vi "Model Initial Values - Add Models RTM Dependency.vi"(8 "error in (no error)":errorcluster, 9 "Menu hierarchy in":string[](array[string]), 11 "Node Ptr":u64 format="%.0x") -> (0 "error out":errorcluster, 1 "Menu hierarchy out":string[](array[string]), 3 "Action":T1)   [LabVIEW 2011, in "Model Initial Values Custom Device.lvlib"]
uses:
  Model Initial Values Custom Device.lvlib
  <vilib>/NI Veristand/Custom Device API/Custom Device RTM Dependency.ctl
  Model Initial Values - Global.vi
  <vilib>/NI Veristand/Custom Device API/Get Item Property (Dependent Node Pointer).vi
  <vilib>/NI Veristand/Custom Device API/Custom Device API.lvlib
  <vilib>/NI Veristand/Custom Device Tools/Custom Device Utility Library/Custom Device Utility Library.lvlib
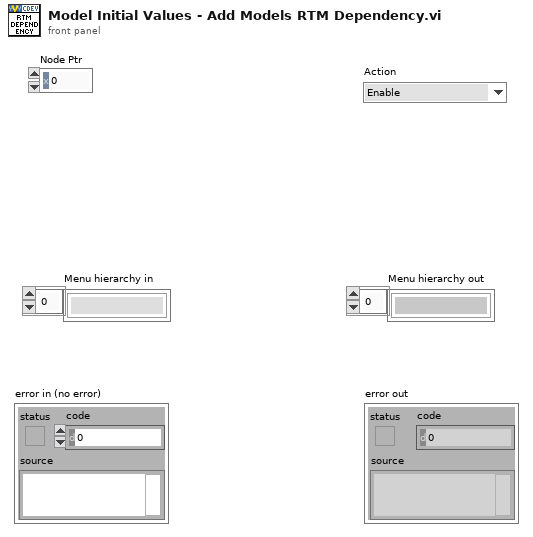
[diagram p1: front panel]
types:
  T1 = typedef "Custom Device API.lvlib/Custom Device RTM Dependency.ctl" = enum16{"Enable", "Disable", "Hide"}
  T2 = typedef "Custom Device API.lvlib/Custom Device Item Ref.ctl" = u64
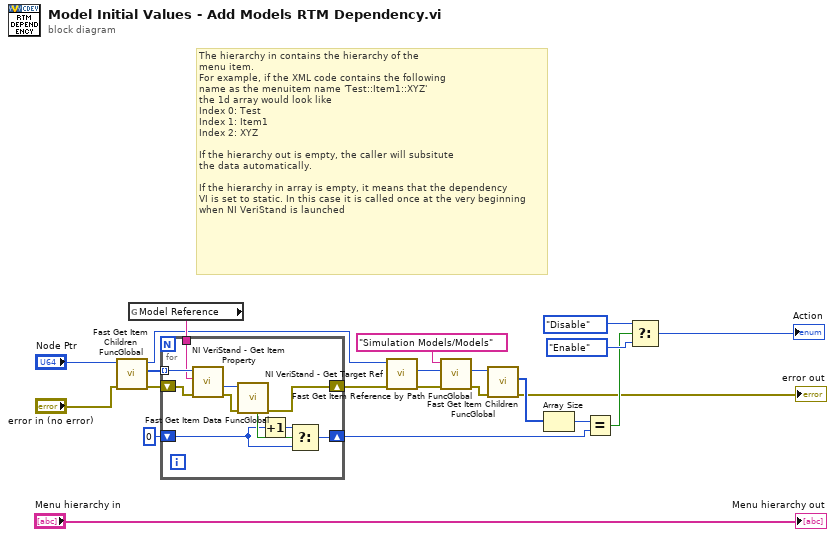
[diagram p0: block diagram]
diagram:
  # "The hierarchy in contains the hierarchy of the\nmenu item.\nFor example, if the XML code contains the following\nname as the menuitem name 'Test::Item1::XYZ'\nthe 1d array would look like\nIndex 0: Test\nIndex 1: Item1\nIndex 2: XYZ\n\nIf the hierarchy out is empty, the caller will subsitute\nthe data automatically.\n\nIf the hierarchy in array is empty, it means that the dependency\nVI is set to static. In this case it is called once at the very beginning\nwhen NI VeriStand is launched"
  n1 = call "Fast Get Item Children FuncGlobal.vi"("error in (no error)"="error in (no error)", "Item Ref in"="Node Ptr") -> ("error out"=w15:errorcluster, "Child Refs"=w16:T2[], "Item Ref out"=w8:T2)  [unwired: 6 in, 1 out]
  n2 = global read "Model Initial Values - Global.vi" "Model Reference"() -> (w14:string)
  n3 = for {
    tunnel: w16 -> [w31] mode=indexing
    shift-right: [w23] -> w9
    shift-left: w15 -> [w29]
    tunnel: w14 -> [w28]
    shift-right: [w25] -> w3
    shift-left: 0 -> [w24]
    n4 = call-poly <vilib>:"NI VeriStand - Get Item Property.vi"("error in (no error)"=w29, "Property Name"=w28, "Item Ref in"=w31) -> ("error out"=w30:errorcluster, "Dependent Node Ref"=w32:T2)  [unwired: 5 in, 2 out]
    n5 = call "Fast Get Item Data FuncGlobal.vi"("error in (no error)"=w30, "Item Ref in"=w32) -> ("error out"=w23:errorcluster, "Found"=w26:bool)  [unwired: 6 in, 2 out]
    n6 = Increment(x=w24) -> (x+1=w27:i32)
    n7 = Select(t=w27, s=w26, f=w24) -> (s? t:f=w25:i32)
  }
  n8 = call <vilib>:"NI VeriStand - Get Target Ref.vi"("error in"=w9, "Item Ref in"=w8) -> ("error out"=w10:errorcluster, "Target Ref"=w12:T2)  [unwired: 6 in, 2 out]
  n9 = call "Fast Get Item Reference by Path FuncGlobal.vi"("error in (no error)"=w10, "Root Ref"=w12, "Item Path in"="Simulation Models/Models" ("Relative Item Path")) -> ("error out"=w6:errorcluster, "Item Ref"=w7:T2)  [unwired: 5 in, 2 out]
  n10 = call "Fast Get Item Children FuncGlobal.vi"("error in (no error)"=w6, "Item Ref in"=w7) -> ("error out"=→"error out":errorcluster, "Child Refs"=w5:T2[])  [unwired: 6 in, 2 out]
  n11 = Array Size(array=w5) -> (size(s)=w4:i32)
  n12 = Equal?(x=w4, y=w3) -> (x = y?=w2:bool)
  n13 = Select(t=Custom_Device_RTM_Dependency."Disable" ("Action"), s=w2, f=Custom_Device_RTM_Dependency."Enable" ("Action")) -> (s? t:f=→"Action":T1)
  "Menu hierarchy out" <- "Menu hierarchy in"
